vi "ExposeMapperGetValueNamepathDescription.vi"(9 "ColRefVals":bool caption="Collect reference values (f)\n(Will need deletion!!)", 10 "Namepath Info":T3, 11 "Data Value Reference in":refnum<data-value>) -> (1 "Controls Found":refnum<vi>[](array[refnum]), 2 "NPDsc":T1[](array[typedef]) caption="Namepath Desription", 3 "Data Value Refrence out":refnum<data-value>)   [LabVIEW 2017]
uses:
  ExposeObjectMapNamepathData.ctl
  ExposeMapperDataTypeEnum.ctl
  ExposeObjectMapContainerTypeEnum.ctl
  ExposeMapperUpdateNamepathPartDescriptor.ctl
  ExposeMapperUpdateNamepathPartDescriptorEnum.ctl
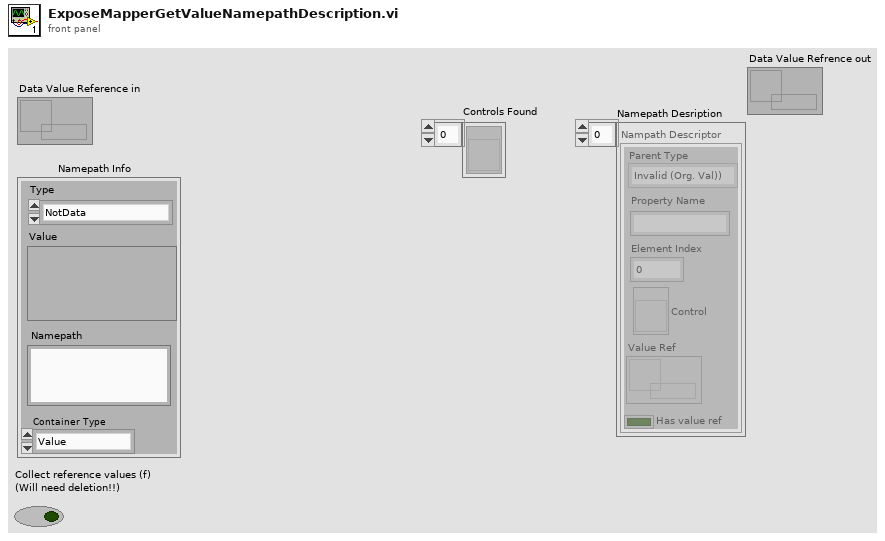
[diagram p1: front panel]
types:
  T1 = typedef "ExposeMapperUpdateNamepathPartDescriptor.ctl" = cluster{"Parent Type":T2, "Property Name":string, "Element Index":i32, "Control":refnum<vi>, "Value Ref":refnum<data-value>, "Has value ref":bool}
  T2 = typedef "ExposeMapperUpdateNamepathPartDescriptorEnum.ctl" = enum16{"Invalid (Org. Val))", "Default Value", "Value", "Variant", "Cluster", "Array", "Refnum"}
  T3 = typedef "ExposeObjectMapNamepathData.ctl" = cluster{"Type":T4, "Value":variant, "Namepath":string, "Container Type":T5}
  T4 = typedef "ExposeMapperDataTypeEnum.ctl" = enum16{"NotData", "int8", "byte", "int16", "uint16", "int32", "uint32", "int64", "uint64", "Single", "Double", "String", "Boolean", "Container"}
  T5 = typedef "ExposeObjectMapContainerTypeEnum.ctl" = enum16{"Value", "Array", "Waveform", "NetContainer"}
  T6 = typedef "ExposeMapperObjectTypeEnum.ctl" = enum16{"NotAValidObject", "Value", "Variant", "Cluster", "Array", "Asng. Refnum"}
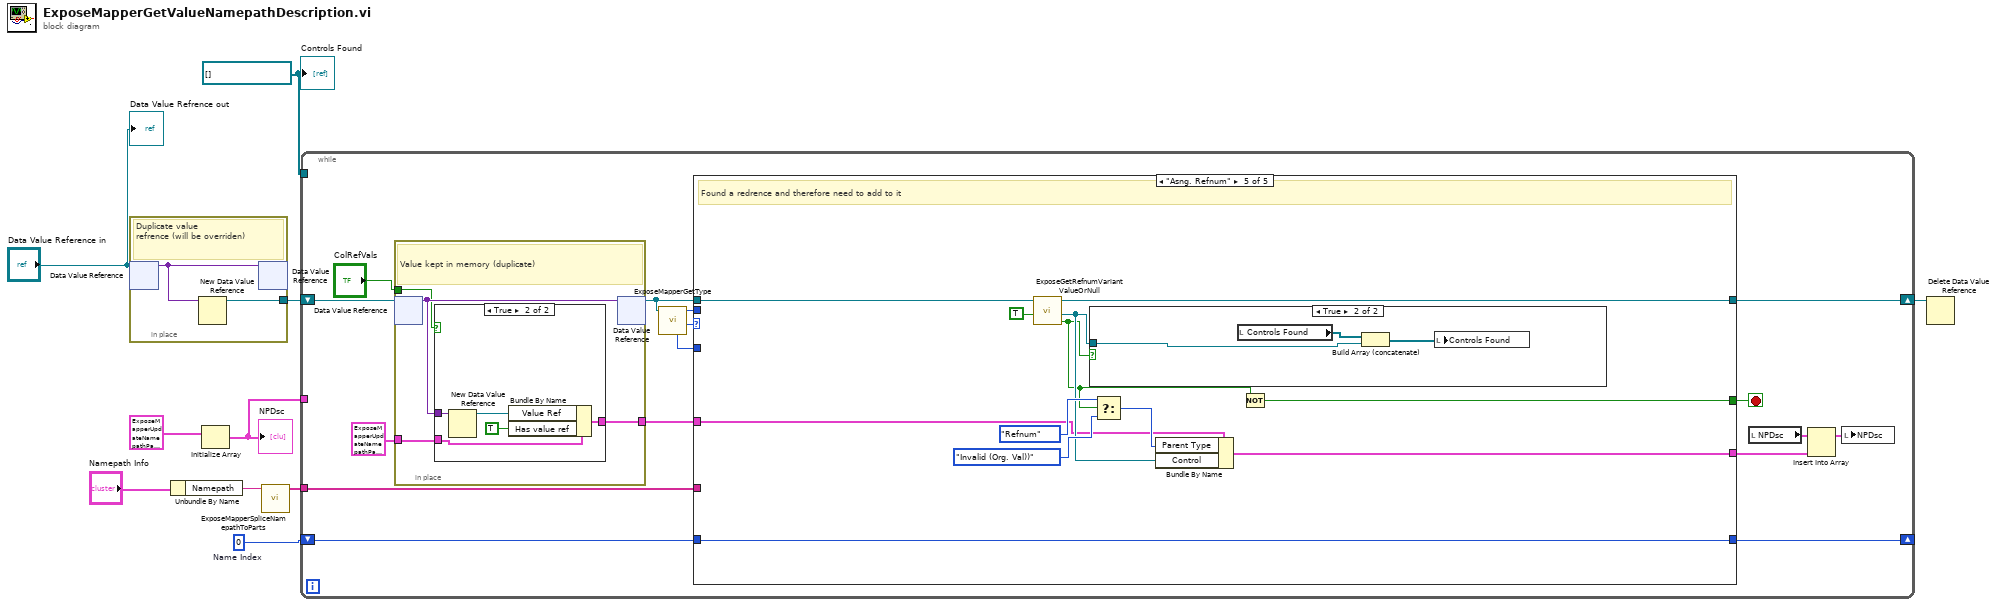
[diagram p0: block diagram]
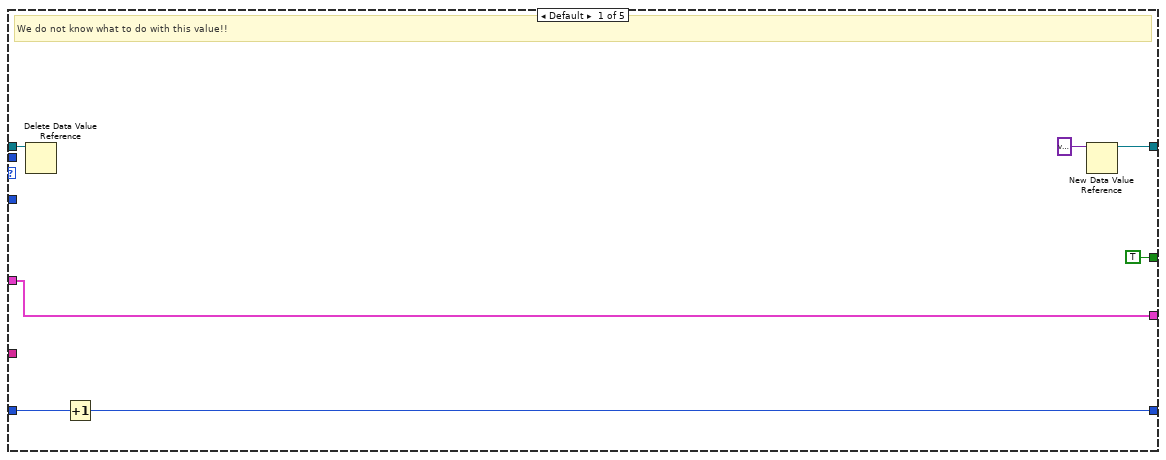
[diagram p2: hidden frame]
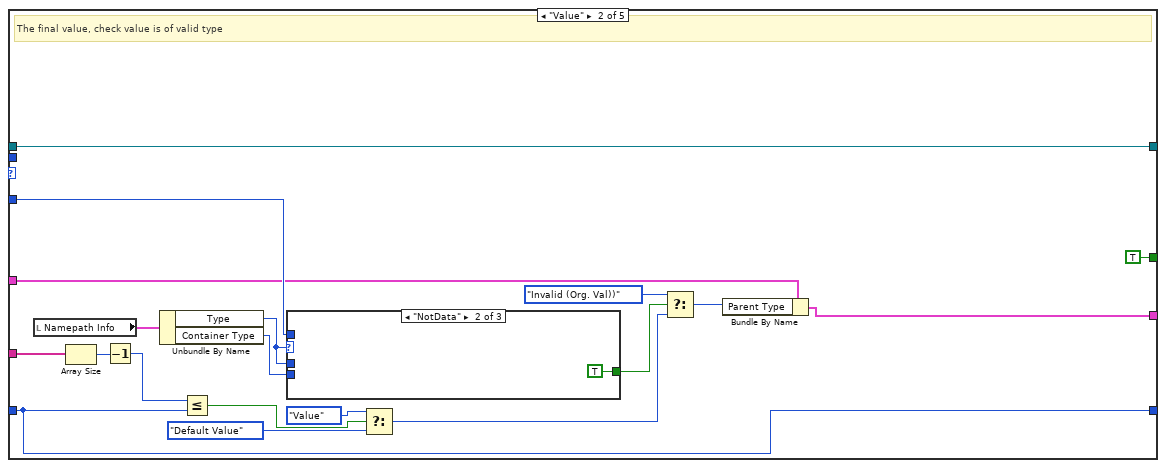
[diagram p3: hidden frame]
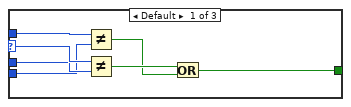
[diagram p4: hidden frame]
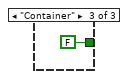
[diagram p5: hidden frame]
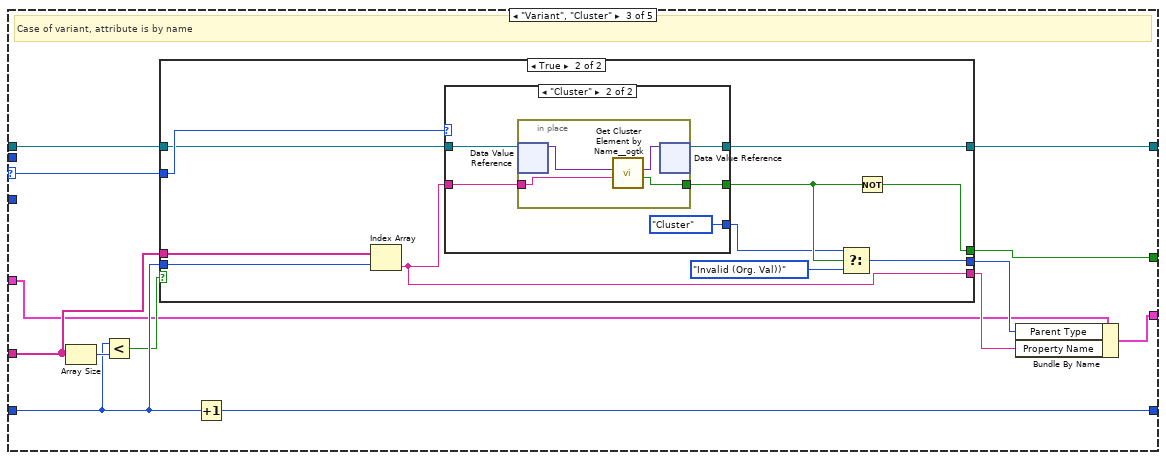
[diagram p6: hidden frame]
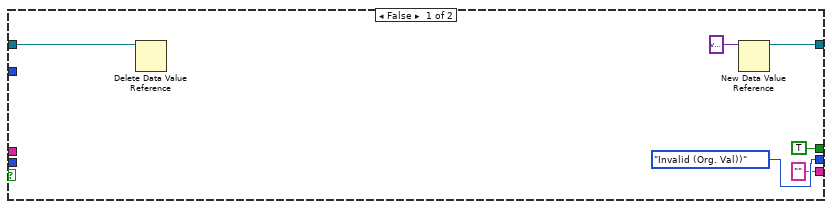
[diagram p7: hidden frame]
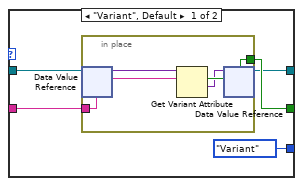
[diagram p8: hidden frame]
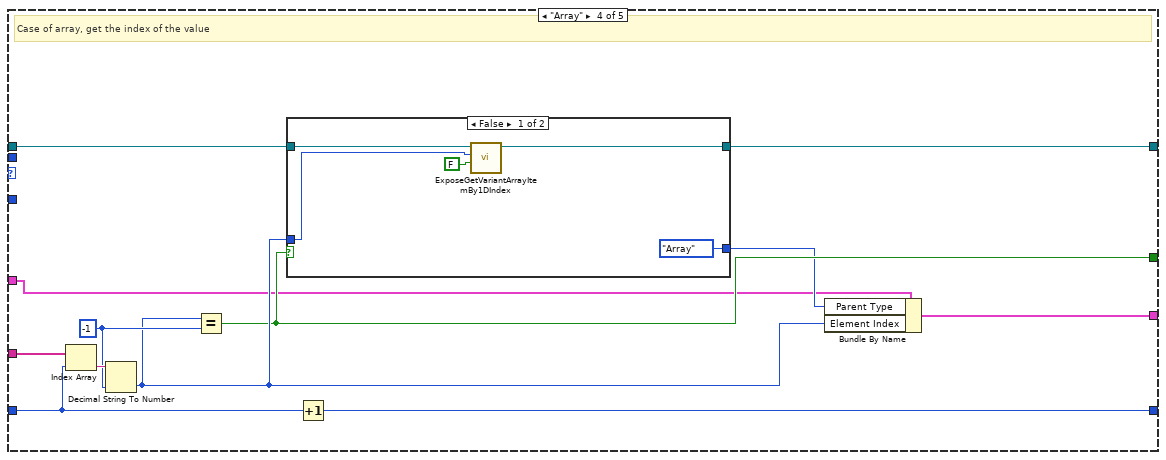
[diagram p9: hidden frame]
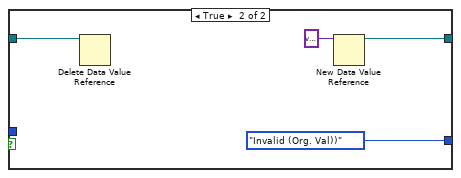
[diagram p10: hidden frame]
diagram:
  w6 = 0  # Name Index
  w4 = refnum<vi>[] [] ("Controls Found")
  n1 = in-place {
    in-place-border: [w12] -> w2
    # "Duplicate value \nrefrence (will be overriden)"
    n2 = in-place-dvr #1("Data Value Reference in") -> (w11:variant)  [unwired: 1 out]
    n3 = New Data Value Reference(data value=w11) -> (data value reference=w12:refnum<data-value>)  [unwired: 1 in, 1 out]
    n4 = in-place-dvr #1(w11) -> ()  [unwired: 2 out]
  }
  n5 = Unbundle By Name("Namepath Info") -> ("Namepath"=w9:string)
  n6 = Initialize Array(T1 {"Parent Type"=enum."Invalid (Org. Val))", "Property Name"="", "Element Index"=0, "Control"=refnum, "Value Ref"=refnum, "Has value ref"=FALSE} ("Nampath Descriptor")) -> (w5:T1[])  [unwired: 1 in]
  "NPDsc" <- w5
  n7 = call "ExposeMapperSpliceNamepathToParts.vi"("Namepath"=w9) -> ("Array of Strings"=w8:string[])  [unwired: 10 in]
  n8 = while {
    shift-right: [w17] -> w1
    shift-left: w2 -> [w21]
    tunnel: w8 -> [w27]
    shift-right: [w28] -> _
    shift-left: w6 -> [w26]
    tunnel: w5 -> [_]
    tunnel: w4 -> [_]
    stop <- w25 stop-if-true
    n9 = in-place {
      in-place-border: T1 {"Parent Type"=enum."Invalid (Org. Val))", "Property Name"="", "Element Index"=0, "Control"=refnum, "Value Ref"=refnum, "Has value ref"=FALSE} ("Nampath Descriptor") -> [w150]
      in-place-border: [w151] -> w19
      in-place-border: "ColRefVals" -> [w148]
      # "Value kept in memory (duplicate)"
      n10 = in-place-dvr #2(w21) -> (w149:variant)  [unwired: 1 out]
      n11 = case shown="True" w148 {
        tunnel: w149 -> [_ w157]
        tunnel: [w152 w155] -> w151
        tunnel: w150 -> [w152 w154]
        frame False {
        }
        frame True {
          n12 = New Data Value Reference(data value=w157) -> (data value reference=w153:refnum<data-value>)  [unwired: 1 in, 1 out]
          n13 = Bundle By Name(cluster=w154, "Value Ref"=w153, "Has value ref"=TRUE) -> (w155:T1)
        }
      }
      n14 = in-place-dvr #2(w149) -> (w13:refnum<data-value>)  [unwired: 1 out]
    }
    n15 = call "ExposeMapperGetType.vi"("Data Val Ref in"=w13) -> ("OType"=w16:T6, "DataType"=w15:T4, "Container Type (Labview Value type)"=w14:T5)  [unwired: 5 in, 3 out]
    n16 = case shown="\"Asng. Refnum\"" w16 {
      selector: w16 -> [_ _ w67 _ _]
      tunnel: [w33 w44 w72 w123 w144] -> w28
      tunnel: w26 -> [w34 w44 w69 w121 w144]
      tunnel: [w29 w50 w76 w118 w143] -> w22
      tunnel: [TRUE TRUE w75 w116 w142] -> w25
      tunnel: w27 -> [_ w45 w71 w122 _]
      tunnel: w15 -> [_ _ _ _ _]
      tunnel: w14 -> [_ w40 _ _ _]
      tunnel: w19 -> [w29 w39 w66 w112 w136]
      tunnel: w13 -> [w32 w42 w65 w114 w133]
      tunnel: [w30 w42 w64 w113 w134] -> w17
      frame Default {
        # "We do not know what to do with this value!!"
        n17 = Delete Data Value Reference(data value reference=w32) -> ()  [unwired: 1 in, 2 out]
        n18 = Increment(x=w34) -> (x+1=w33:i32)
        n19 = New Data Value Reference(data value=variant ("Value")) -> (data value reference=w30:refnum<data-value>)  [unwired: 1 in, 1 out]
      }
      frame "Value" {
        # "The final value, check value is of valid type"
        n20 = local read "Namepath Info"() -> (w38:T3)
        n21 = Array Size(array=w45) -> (size(s)=w54:i32)
        n22 = Decrement(x=w54) -> (x-1=w43:i32)
        n23 = Unbundle By Name(w38) -> ("Type"=w36:T4, "Container Type"=w37:T5)
        n24 = Less Or Equal?(x=w43, y=w44) -> (x <= y?=w53:bool)
        n25 = case shown="\"NotData\"" w36 {
          selector: w36 -> [w59 _ _]
          tunnel: [w61 TRUE FALSE] -> w41
          tunnel: w40 -> [w60 _ _]
          tunnel: w36 -> [w56 _ _]
          tunnel: w37 -> [w55 _ _]
          frame Default {
            n26 = Not Equal?(x=w60, y=w55) -> (x != y?=w57:bool)
            n27 = Not Equal?(x=w59, y=w56) -> (x != y?=w58:bool)
            n28 = Or(x=w58, y=w57) -> (x .or. y?=w61:bool)
          }
          frame "NotData" {
          }
          frame "Container" {
          }
        }
        n29 = Select(t=ExposeMapperUpdateNamepathPartDescriptorEnum."Value" ("Update Type"), s=w53, f=ExposeMapperUpdateNamepathPartDescriptorEnum."Default Value" ("Update Type")) -> (s? t:f=w47:T2)
        n30 = Select(t=ExposeMapperUpdateNamepathPartDescriptorEnum."Invalid (Org. Val))" ("Update Type"), s=w41, f=w47) -> (s? t:f=w46:T2)
        n31 = Bundle By Name(cluster=w39, "Parent Type"=w46) -> (w50:T1)
      }
      frame "Variant", "Cluster" {
        # "Case of variant, attribute is by name"
        n32 = Array Size(array=w71) -> (size(s)=w70:i32)
        n33 = Less?(x=w69, y=w70) -> (x < y?=w68:bool)
        n34 = case shown="True" w68 {
          tunnel: [TRUE w92] -> w75
          tunnel: [ExposeMapperUpdateNamepathPartDescriptorEnum."Invalid (Org. Val))" ("Update Type") w90] -> w74
          tunnel: ["" w86] -> w73
          tunnel: w71 -> [_ w89]
          tunnel: w69 -> [_ w88]
          tunnel: w67 -> [_ w87]
          tunnel: w65 -> [w79 w84]
          tunnel: [w77 w83] -> w64
          frame False {
            n35 = Delete Data Value Reference(data value reference=w79) -> ()  [unwired: 1 in, 2 out]
            n36 = New Data Value Reference(data value=variant ("VElement")) -> (data value reference=w77:refnum<data-value>)  [unwired: 1 in, 1 out]
          }
          frame True {
            n37 = Index Array(array=w89, index=w88) -> (element=w86:string)
            n38 = case shown="\"Cluster\"" w87 {
              tunnel: [w98 w103] -> w91
              tunnel: w86 -> [w97 w107]
              tunnel: [ExposeMapperUpdateNamepathPartDescriptorEnum."Variant" ("Update Type") ExposeMapperUpdateNamepathPartDescriptorEnum."Cluster" ("Update Type")] -> w85
              tunnel: w84 -> [w95 w105]
              tunnel: [w94 w104] -> w83
              frame "Variant", Default {
                n39 = in-place {
                  in-place-border: [w102] -> w98
                  in-place-border: w97 -> [w101]
                  n40 = in-place-dvr #3(w95) -> (w100:variant)  [unwired: 1 out]
                  n41 = Get Variant Attribute(Variant=w100, name=w101) -> (found=w102:bool, value=w99:variant)  [unwired: 2 in, 2 out]
                  n42 = in-place-dvr #3(w99) -> (w94:refnum<data-value>)  [unwired: 1 out]
                }
              }
              frame "Cluster" {
                n43 = in-place {
                  in-place-border: w107 -> [w110]
                  in-place-border: [w108] -> w103
                  n44 = in-place-dvr #4(w105) -> (w111:variant)  [unwired: 1 out]
                  n45 = call <userlib>:"Get Cluster Element by Name__ogtk.vi"("Element Name"=w110, "Cluster"=w111) -> ("found?"=w108:bool, "VElement"=w109:variant)  [unwired: 7 in, 1 out]
                  n46 = in-place-dvr #4(w109) -> (w104:refnum<data-value>)  [unwired: 1 out]
                }
              }
            }
            n47 = Select(t=w85, s=w91, f=ExposeMapperUpdateNamepathPartDescriptorEnum."Invalid (Org. Val))" ("Update Type")) -> (s? t:f=w90:T2)
            n48 = Not(x=w91) -> (.not. x?=w92:bool)
          }
        }
        n49 = Increment(x=w69) -> (x+1=w72:i32)
        n50 = Bundle By Name(cluster=w66, "Parent Type"=w74, "Property Name"=w73) -> (w76:T1)
      }
      frame "Array" {
        w119 = -1 ("default (0 I32)")
        # "Case of array, get the index of the value"
        n51 = Index Array(array=w122, index=w121) -> (element=w120:string)
        n52 = Decimal String To Number(string=w120, default (0L)=w119) -> (number=w117:i32)  [unwired: 1 in, 1 out]
        n53 = Equal?(x=w117, y=w119) -> (x = y?=w116:bool)
        n54 = case shown="False" w116 {
          tunnel: w117 -> [w128 _]
          tunnel: [ExposeMapperUpdateNamepathPartDescriptorEnum."Array" ("Update Type") ExposeMapperUpdateNamepathPartDescriptorEnum."Invalid (Org. Val))" ("Update Type")] -> w115
          tunnel: w114 -> [w125 w131]
          tunnel: [w124 w129] -> w113
          frame False {
            n55 = call "ExposeGetVariantArrayItemBy1DIndex.vi"("Pad if dose not exist? (t)"=FALSE, "Index"=w128, "Array Reference in"=w125) -> ("Array Reference Out"=w124:refnum<data-value>)  [unwired: 7 in, 1 out]
          }
          frame True {
            n56 = Delete Data Value Reference(data value reference=w131) -> ()  [unwired: 1 in, 2 out]
            n57 = New Data Value Reference(data value=variant ("Array Element")) -> (data value reference=w129:refnum<data-value>)  [unwired: 1 in, 1 out]
          }
        }
        n58 = Increment(x=w121) -> (x+1=w123:i32)
        n59 = Bundle By Name(cluster=w112, "Parent Type"=w115, "Element Index"=w117) -> (w118:T1)
      }
      frame "Asng. Refnum" {
        # "Found a redrence and therefore need to add to it"
        n60 = call "ExposeGetRefnumVariantValueOrNull.vi"("Get default value ? (f)"=TRUE, "Data Value Reference in"=w133) -> ("IsControl"=w137:bool, "Control"=w138:refnum<vi>, "Data Value Reference Out"=w134:refnum<data-value>)  [unwired: 7 in]
        n61 = case shown="True" w137 {
          tunnel: w138 -> [_ w146]
          frame False {
          }
          frame True {
            n62 = local read "Controls Found"() -> (w147:refnum<vi>[])
            n63 = Build Array (concatenate)(w147, w146) -> (w145:refnum<vi>[])
            n64 = local write "Controls Found"(w145) -> ()
          }
        }
        n65 = Select(t=ExposeMapperUpdateNamepathPartDescriptorEnum."Refnum" ("Update Type"), s=w137, f=ExposeMapperUpdateNamepathPartDescriptorEnum."Invalid (Org. Val))" ("Update Type")) -> (s? t:f=w139:T2)
        n66 = Bundle By Name(cluster=w136, "Parent Type"=w139, "Control"=w138) -> (w143:T1)
        n67 = Not(x=w137) -> (.not. x?=w142:bool)
      }
    }
    n68 = local read "NPDsc"() -> (w23:T1[])
    n69 = Insert Into Array(array=w23, new element=w22) -> (w24:T1[])  [unwired: 1 in]
    n70 = local write "NPDsc"(w24) -> ()
  }
  n71 = Delete Data Value Reference(data value reference=w1) -> ()  [unwired: 1 in, 2 out]
  "Controls Found" <- w4
  "Data Value Refrence out" <- "Data Value Reference in"
